vi "Multiple Connections - Client Tx1.vi"() -> ()   [LabVIEW 2011]
doc: "Establishes a connection to the specified host and port and reads the date and time data sent by the Server. It first reads 4 bytes defining the length of the date & time string and then reads the data. After you click the stop button, this VI sends a single character to tell the Date Server VI to terminate the connection.\n\n<B>Note:</B> Requires the use of the Multiple Connections - Server.vi."
panel:
  in  "data in":string="12345:67890"
  in  "Send":bool
  in  "stop":bool
  in  "Machine":string="localhost"
  in  "Port":u16=6341
  # "Instructions:\n1. Open the Multiple Connections - Server.vi.\n2. Run the Multiple Connections - Server.vi first.\n3. Run the Client VIs second.\n4. Stop this VI and restart it to notice the # of Connections on the Server VI change.\n5. Stop the Server VI.  This VI will stop when it times out."
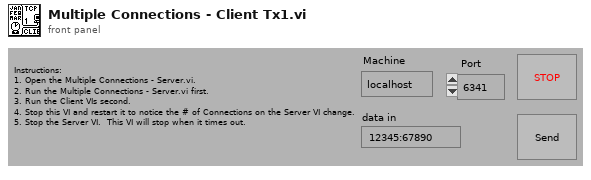
[diagram p1: front panel]
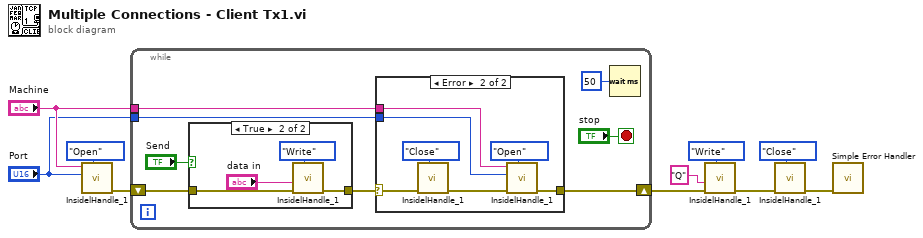
[diagram p0: block diagram]
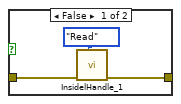
[diagram p2: hidden frame]
diagram:
  n1 = call "InsidelHandle_1.vi"("Mode"=enum16{"Open", "Read", "Write", "Close"}."Open", "Port"="Port", "Machine"="Machine") -> ("error out"=w9:errorcluster)  [unwired: 7 in, 1 out]
  n2 = while {
    shift-right: [w17] -> w5
    shift-left: w9 -> [w16]
    tunnel: "Machine" -> [w14]
    tunnel: "Port" -> [w13]
    stop <- "stop" stop-if-true
    n3 = case shown="True" "Send" {
      tunnel: w16 -> [w20 w25]
      tunnel: [w19 w24] -> w15
      frame False {
        n4 = call "InsidelHandle_1.vi"("Mode"=enum16{"Open", "Read", "Write", "Close"}."Read", "error in (no error)"=w20) -> ("error out"=w19:errorcluster)  [unwired: 8 in, 1 out]
      }
      frame True {
        n5 = call "InsidelHandle_1.vi"("Mode"=enum16{"Open", "Read", "Write", "Close"}."Write", "error in (no error)"=w25, "data in"="data in") -> ("error out"=w24:errorcluster)  [unwired: 7 in, 1 out]
      }
    }
    n6 = case shown="Error" w15 {
      selector: w15 -> [w26 w29]
      tunnel: [w26 w30] -> w17
      tunnel: w14 -> [_ w28]
      tunnel: w13 -> [_ w27]
      frame No Error {
      }
      frame Error {
        n7 = call "InsidelHandle_1.vi"("Mode"=enum16{"Open", "Read", "Write", "Close"}."Close", "error in (no error)"=w29) -> ("error out"=w31:errorcluster)  [unwired: 8 in, 1 out]
        n8 = call "InsidelHandle_1.vi"("Mode"=enum16{"Open", "Read", "Write", "Close"}."Open", "error in (no error)"=w31, "Port"=w27, "Machine"=w28) -> ("error out"=w30:errorcluster)  [unwired: 6 in, 1 out]
      }
    }
    n9 = Wait (ms)(milliseconds to wait=u32 50) -> ()  [unwired: 1 out]
  }
  n10 = call "InsidelHandle_1.vi"("Mode"=enum16{"Open", "Read", "Write", "Close"}."Write", "error in (no error)"=w5, "data in"="Q") -> ("error out"=w6:errorcluster)  [unwired: 7 in, 1 out]
  n11 = call "InsidelHandle_1.vi"("Mode"=enum16{"Open", "Read", "Write", "Close"}."Close", "error in (no error)"=w6) -> ("error out"=w1:errorcluster)  [unwired: 8 in, 1 out]
  n12 = call <vilib>:"Simple Error Handler.vi"("error in (no error)"=w1) -> ()  [unwired: 1 in, 8 out]
